vi "Initiate Pulse Test Dual.vi"(7 "Timeout (10000 ms)":u32=10000, 8 "error in":errorcluster, 9 "Tag 2":u32=2, 10 "Tag 1":u32=1, 11 "VISA resource name":refnum<visa-resource-name>) -> (0 "error out":errorcluster, 1 "Message":string, 2 "Success":bool, 3 "VISA resource name out":refnum<visa-resource-name>, 4 "Command String":string)   [LabVIEW 2013, in "Keithley 2600 Series.lvlib"]
doc: "This VI will instruct the instrument to initiate the output of two pre-configured pulse trains.\n\n<b>Remarks:</b>\n• <b>Tag 1</b> and <b>Tag 2</b> may not be the same number.\n• The configured pulses referenced by the tags must be for different channels.\n\n<b>Functions and Attributes Used</b>\nInititatePulseTestDual(tag1, tag2)"
uses:
  Keithley 2600 Series.lvlib
  Private/GlobalVariables.vi
panel:
  # "(c) 2008 Keithley Instruments, Inc.  ALL RIGHTS RESERVED."
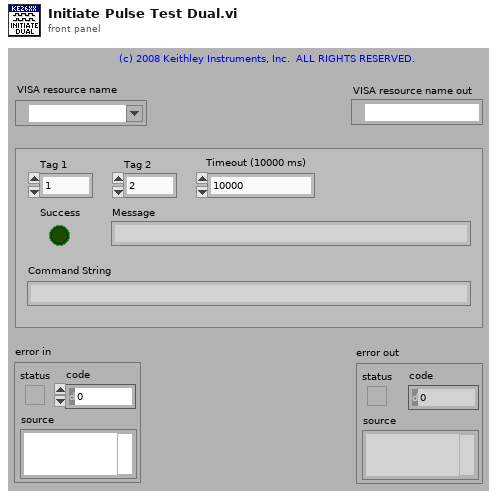
[diagram p1: front panel]
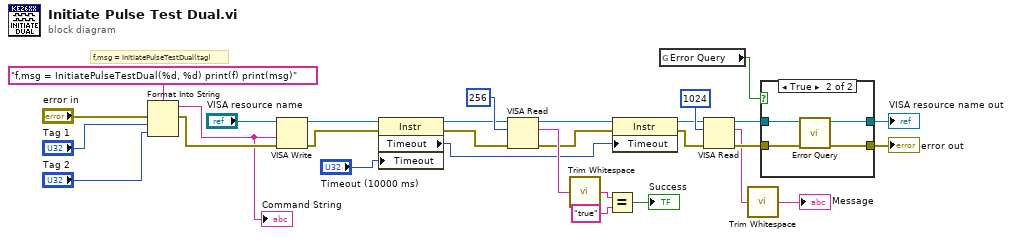
[diagram p0: block diagram]
diagram:
  # "f,msg = InitiatePulseTestDual(tag)"
  n1 = Format Into String(format string="f,msg = InitiatePulseTestDual(%d, %d) print(f) print(msg)", error in="error in", "Tag 1", "Tag 2") -> (resulting string=w20:string, error out=w26:errorcluster)  [unwired: 1 in]
  "Command String" <- w20
  n2 = VISA Write(VISA resource name="VISA resource name", write buffer=w20, error in (no error)=w26) -> (VISA resource name out=w10:refnum<visa-resource-name>, error out=w9:errorcluster)  [unwired: 1 out]
  n3 = property class="Instr"(reference=w10, error in=w9, "Timeout"="Timeout (10000 ms)") -> (reference out=w7:refnum<visa-resource-name>, error out=w6:errorcluster, "Timeout"=w1:u32)
  n4 = VISA Read(VISA resource name=w7, byte count=u32 256, error in (no error)=w6) -> (VISA resource name out=w2:refnum<visa-resource-name>, read buffer=w14:string, error out=w3:errorcluster)  [unwired: 1 out]
  n5 = call <vilib>:"Trim Whitespace.vi"("string"=w14) -> ("trimmed string"=w16:string)  [unwired: 1 in]
  n6 = Equal?(x=w16, y="true") -> (x = y?=→"Success":bool)
  n7 = property class="Instr"(reference=w2, error in=w3, "Timeout"=w1) -> (reference out=w5:refnum<visa-resource-name>, error out=w4:errorcluster)
  n8 = global read "GlobalVariables.vi" "Error Query"() -> (w25:bool)
  n9 = VISA Read(VISA resource name=w5, byte count=u32 1024, error in (no error)=w4) -> (VISA resource name out=w18:refnum<visa-resource-name>, read buffer=w13:string, error out=w19:errorcluster)  [unwired: 1 out]
  n10 = call <vilib>:"Trim Whitespace.vi"("string"=w13) -> ("trimmed string"=→"Message":string)  [unwired: 1 in]
  n11 = case shown="True" w25 {
    tunnel: [w32 w36] -> w22
    tunnel: [w31 w35] -> w21
    tunnel: w18 -> [w32 w34]
    tunnel: w19 -> [w31 w33]
    frame False {
    }
    frame True {
      n12 = call "Error Query.vi"("error in (no error)"=w33, "VISA resource name"=w34) -> ("error out"=w35:errorcluster, "VISA resource name out"=w36:refnum<visa-resource-name>)  [unwired: 8 out]
    }
  }
  "VISA resource name out" <- w22
  "error out" <- w21
